vi "Initialize.vi"(5 "components directory (default)":path, 7 "framework options":T1, 8 "error in (no error)":errorcluster, 10 "framework configuration":T6, 11 "Framework in":refnum<class "Framework.lvclass">) -> (0 "error out":errorcluster, 3 "Framework out":refnum<class "Framework.lvclass">)   [LabVIEW 2017, in "DSF Core.lvlib" / "Framework.lvclass"]
uses:
  Framework.lvclass
  Typedefs/DSF Engine Framework Configuration.ctl
  Typedefs/DSF Engine Plugin Configuration.ctl
  Typedefs/DSF Timing Info.ctl
  Typedefs/DSF Engine Plugin Thread Configuration.ctl
  Typedefs/DSF Settings Info.ctl
  Typedefs/DSF Engine Transfer Group Configuration.ctl
  Typedefs/DSF Direction.ctl
  Typedefs/DSF Engine Transfer Configuration.ctl
  Typedefs/DSF Byte Order.ctl
  Typedefs/DSF Engine Channel Configuration.ctl
  Typedefs/DSF Data Type.ctl
  Typedefs/DSF Timeout Behavior.ctl
  Framework Options.ctl
  Typedefs/DSF FIFO Options.ctl
  Thread/DSF Thread Options.ctl
  Typedefs/DSF Plugin Options.ctl
  Typedefs/DSF Performance Options.ctl
  Framework States.ctl
  Thread/Plugin/Plugin Thread.lvclass
  C:/Git/DSF/Core/Classes/Thread/Thread.lvclass
  Thread/Logging/Logging Thread.lvclass
  Thread/Dispatcher/Dispatcher Thread.lvclass
  DSF Core.lvlib
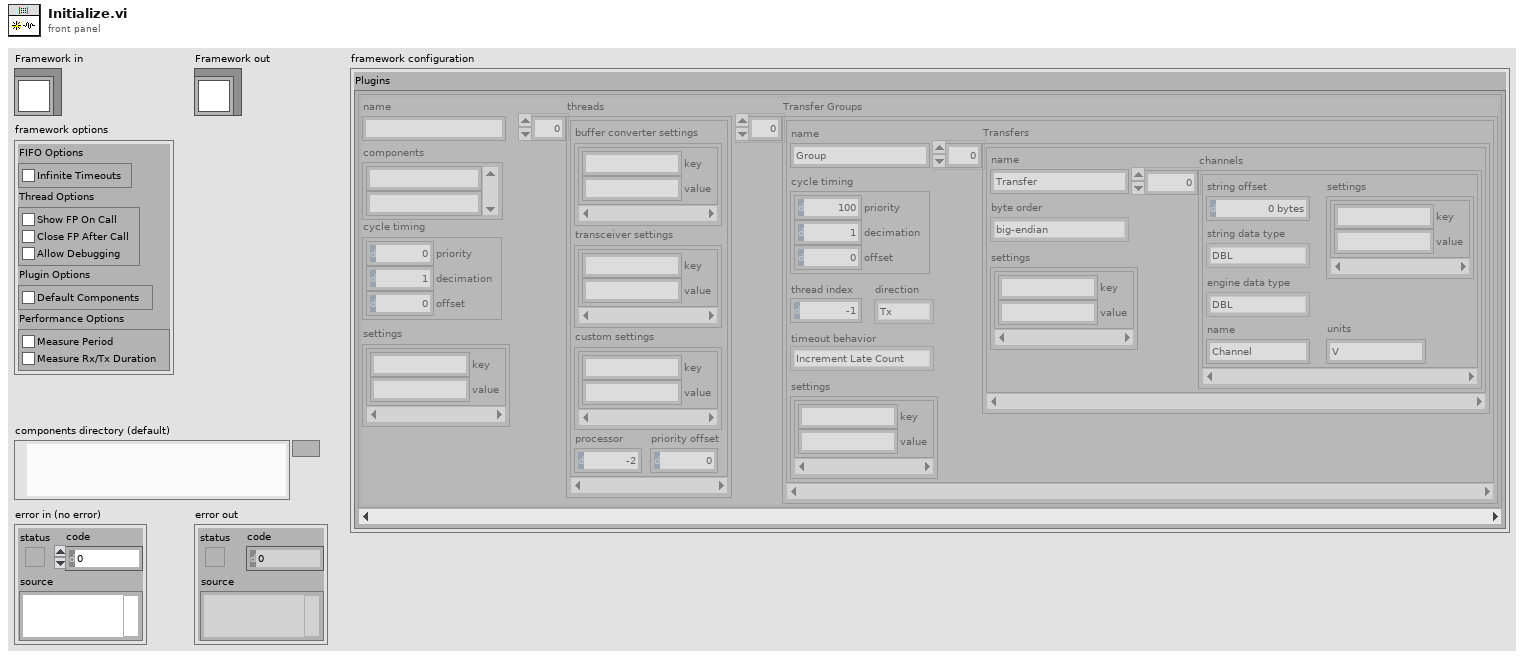
[diagram p1: front panel]
types:
  T1 = typedef "DSF Core.lvlib/Framework.lvclass/Framework Options.ctl" = cluster{"FIFO Options":T2, "Thread Options":T3, "Plugin Options":T4, "Performance Options":T5}
  T2 = typedef "DSF Core.lvlib/DSF FIFO Options.ctl" = cluster{"Infinite Timeouts":bool}
  T3 = typedef "DSF Core.lvlib/DSF Thread Options.ctl" = cluster{"Show FP On Call":bool, "Close FP After Call":bool, "Allow Debugging":bool}
  T4 = typedef "DSF Core.lvlib/DSF Plugin Options.ctl" = cluster{"Default Components":bool}
  T5 = typedef "DSF Core.lvlib/DSF Performance Options.ctl" = cluster{"Measure Period":bool, "Measure Rx/Tx Duration":bool}
  T6 = typedef "DSF Core.lvlib/DSF Engine Framework Configuration.ctl" = cluster{"Plugins":T7[]}
  T7 = typedef "DSF Core.lvlib/DSF Engine Plugin Configuration.ctl" = cluster{"name":string, "components":string[], "cycle timing":T8, "threads":T9[], "Transfer Groups":T11[], "settings":T10}
  T8 = typedef "DSF Core.lvlib/DSF Timing Info.ctl" = cluster{"priority":u64, "decimation":u64, "offset":u64}
  T9 = typedef "DSF Core.lvlib/DSF Engine Plugin Thread Configuration.ctl" = cluster{"buffer converter settings":T10, "transceiver settings":T10, "custom settings":T10, "processor":i32, "priority offset":i16}
  T10 = typedef "DSF Core.lvlib/DSF Settings Info.ctl" = cluster{"key":string, "value":string}[]
  T11 = typedef "DSF Core.lvlib/DSF Engine Transfer Group Configuration.ctl" = cluster{"name":string, "direction":T12, "cycle timing":T8, "thread index":i32, "settings":T10, "Transfers":T13[], "timeout behavior":T17}
  T12 = typedef "DSF Core.lvlib/DSF Direction.ctl" = enum8{"Tx", "Rx"}
  T13 = typedef "DSF Core.lvlib/DSF Engine Transfer Configuration.ctl" = cluster{"name":string, "byte order":T14, "settings":T10, "channels":T15[]}
  T14 = typedef "DSF Core.lvlib/DSF Byte Order.ctl" = enum8{"big-endian", "little-endian"}
  T15 = typedef "DSF Core.lvlib/DSF Engine Channel Configuration.ctl" = cluster{"string offset":u64, "string data type":T16, "engine data type":T16, "name":string, "settings":T10, "units":string}
  T16 = typedef "DSF Core.lvlib/DSF Data Type.ctl" = enum8{"Bool", "SGL", "DBL", "I8", "I16", "I32", "I64", "U8", "U16", "U32", "U64"}
  T17 = typedef "DSF Core.lvlib/DSF Timeout Behavior.ctl" = enum8{"Increment Late Count", "Throw Error"}
  T18 = typedef "DSF Core.lvlib/Framework.lvclass/Framework States.ctl" = enum8{"Uninitialized", "Initialized", "Start", "Rx", "Tx", "Shutdown"}
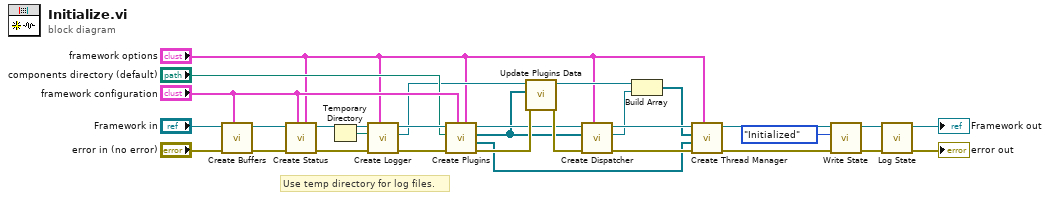
[diagram p0: block diagram]
diagram:
  # "Use temp directory for log files."
  n1 = call "Create Buffers.vi"("framework configuration"="framework configuration", "error in (no error)"="error in (no error)", "Framework in"="Framework in") -> ("error out"=w23:errorcluster, "Framework out"=w24:refnum<class "Framework.lvclass">)  [unwired: 7 in]
  n2 = call "Create Status.vi"("framework options"="framework options", "Framework Configuration"="framework configuration", "error in (no error)"=w23, "Framework in"=w24) -> ("error out"=w18:errorcluster, "Framework out"=w19:refnum<class "Framework.lvclass">)  [unwired: 6 in]
  n3 = Temporary Directory() -> (w14:path)
  n4 = call "Create Logger.vi"("framework options"="framework options", "error in (no error)"=w18, "log file directory"=w14, "Framework in"=w19) -> ("error out"=w16:errorcluster, "Logging Thread"=w12:refnum<class "Logging Thread.lvclass">, "Framework out"=w17:refnum<class "Framework.lvclass">)  [unwired: 4 in, 1 out]
  n5 = call "Create Plugins.vi"("framework options"="framework options", "framework configuration"="framework configuration", "error in (no error)"=w16, "components directory"="components directory (default)", "Framework in"=w17) -> ("error out"=w29:errorcluster, "Plugin Threads"=w9:refnum<class "Plugin Thread.lvclass">[], "Plugins"=w10:refnum<class "Plugin.lvclass">[], "Framework out"=w28:refnum<class "Framework.lvclass">)  [unwired: 3 in]
  n6 = call "Update Plugins Data.vi"("error in (no error)"=w29, "Plugins"=w10, "Logging Thread in"=w12) -> ("error out"=w30:errorcluster, "Logging Thread out"=w11:refnum<class "Logging Thread.lvclass">)  [unwired: 7 in]
  n7 = call "Create Dispatcher.vi"("framework options"="framework options", "error in (no error)"=w30, "Plugins"=w10, "Framework in"=w28) -> ("error out"=w20:errorcluster, "Dispatcher Thread"=w13:refnum<class "Dispatcher Thread.lvclass">, "Framework out"=w22:refnum<class "Framework.lvclass">)  [unwired: 5 in]
  n8 = Build Array(w11, w13) -> (w21:refnum<class "Thread.lvclass">[])
  n9 = call "Create Thread Manager.vi"("framework options"="framework options", "error in (no error)"=w20, "Public Threads"=w9, "Private Threads"=w21, "Framework in"=w22) -> ("error out"=w6:errorcluster, "Framework out"=w7:refnum<class "Framework.lvclass">)  [unwired: 5 in]
  n10 = call "Write State.vi"("error in (no error)"=w6, "state"=Framework_States."Initialized", "Framework in"=w7) -> ("error out"=w3:errorcluster, "Framework out"=w4:refnum<class "Framework.lvclass">)  [unwired: 7 in]
  n11 = call "Log State.vi"("error in (no error)"=w3, "Framework in"=w4) -> ("error out"=→"error out":errorcluster, "Framework out"=→"Framework out":refnum<class "Framework.lvclass">)  [unwired: 8 in]
